vi "Close Sessions.vi"(8 "error in":errorcluster, 11 "session reservation in":refnum<class "Session Reservation.lvclass">) -> (0 "error out":errorcluster, 3 "session reservation out":refnum<class "Session Reservation.lvclass">)   [LabVIEW 2020, in "MeasurementLink Session Management.lvlib" / "Session Reservation.lvclass"]
doc: "Closes all instrument sessions that were created with the session reservation."
uses:
  Session Reservation.lvclass
  Session Reservation.lvclass/Session Reservation.ctl
  MeasurementLink Instrument/IInstrument/IInstrument.lvclass
  MeasurementLink Measurement Server/Helpers/Error Strings Global Internal.vi
  Connection Map/Connection Map.lvclass
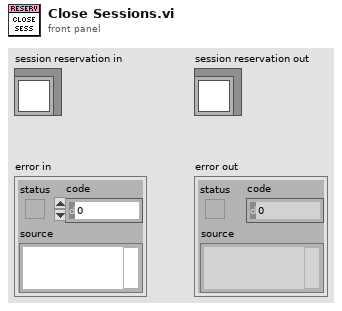
[diagram p1: front panel]
types:
  T1 = typedef "MeasurementLink Session Management.lvlib/Session Reservation.lvclass/Data.ctl" = cluster{"session and driver infos":T2[], "pin or relay names":string[], "connection map":refnum<class "Connection Map.lvclass">, "pin map context":T7, "reservation observer":refnum<class "IReservationObserver.lvclass">, "dvr valid":bool}
  T2 = typedef "MeasurementLink Session Management.lvlib/Session Reservation.lvclass/Session and Driver Info.ctl" = cluster{"session info":T3, "session":variant, "instrument":refnum<class "IInstrument.lvclass">, "initialize and close session behavior":T6}
  T3 = typedef "MeasurementLink Session Management Client.lvlib/ni_measurementlink_sessionmanagement_v1_SessionInformation.ctl" = cluster{"session":T4, "resource_name":string, "channel_list":string, "instrument_type_id":string, "session_exists":bool, "channel_mappings":T5[]}
  T4 = typedef "MeasurementLink Session Management Client.lvlib/nidevice_grpc_Session.ctl" = cluster{"name":string}
  T5 = typedef "MeasurementLink Session Management Client.lvlib/ni_measurementlink_sessionmanagement_v1_ChannelMapping.ctl" = cluster{"pin_or_relay_name":string, "site":i32, "channel":string}
  T6 = typedef "MeasurementLink Instrument.lvlib/IInstrument.lvclass/Initialize and Close Session Behavior.ctl" = enum16{"Create and Close", "Attach and Detach", "Create and Detach", "Attach and Close"}
  T7 = typedef "MeasurementLink Session Management Client.lvlib/ni_measurementlink_PinMapContext.ctl" = cluster{"pin_map_id":string, "sites":i32[]}
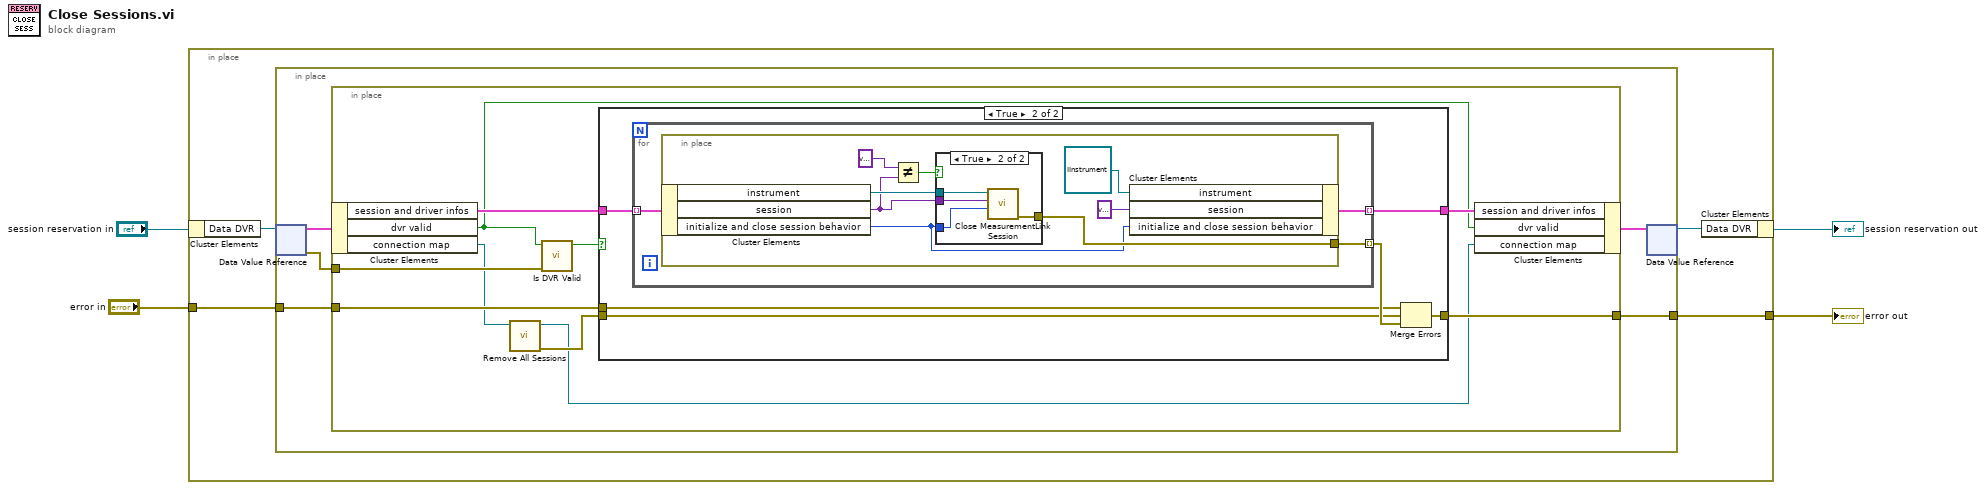
[diagram p0: block diagram]
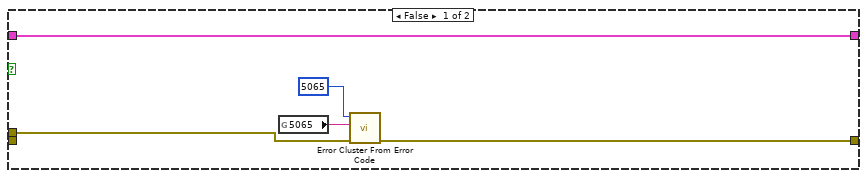
[diagram p2: hidden frame]
diagram:
  n1 = in-place {
    in-place-border: [w6] -> w1
    in-place-border: "error in" -> [w5]
    n2 = in-place-cluster #1("session reservation in") -> ("Data DVR"=w8:refnum<data-value>)
    n3 = in-place {
      in-place-border: [w10] -> w6
      in-place-border: w5 -> [w11]
      n4 = in-place-dvr #2(w8) -> (w12:T1, w13:errorcluster)
      n5 = in-place {
        in-place-border: w13 -> [w23]
        in-place-border: w11 -> [w18]
        in-place-border: [w17] -> w10
        n6 = in-place-cluster #3(w12) -> ("session and driver infos"=w21:T2[], "dvr valid"=w19:bool, "connection map"=w15:refnum<class "Connection Map.lvclass">)
        n7 = call "Remove All Sessions.vi"("connection map in"=w15) -> ("error out"=w16:errorcluster, "connection map out"=w14:refnum<class "Connection Map.lvclass">)  [unwired: 9 in]
        n8 = call "Is DVR Valid.vi"("dvr error in"=w23, "dvr valid"=w19) -> ("dvr valid"=w22:bool)  [unwired: 9 in]
        n9 = case shown="True" w22 {
          tunnel: w21 -> [w28 w34]
          tunnel: [w28 w33] -> w20
          tunnel: w18 -> [w25 w29]
          tunnel: [w24 w32] -> w17
          tunnel: w16 -> [_ w30]
          frame False {
            n10 = global read "Error Strings Global Internal.vi" "5065"() -> (w27:string)
            n11 = call <vilib>:"Error Cluster From Error Code.vi"("error in (no error)"=w25, "error message (\"\")"=w27, "error code (0)"=5065) -> ("error out"=w24:errorcluster)  [unwired: 6 in]
          }
          frame True {
            n12 = for {
              tunnel: w34 -> [w37] mode=indexing
              tunnel: [w36] -> w33 mode=indexing
              tunnel: [w35] -> w31 mode=indexing
              n13 = in-place {
                in-place-border: [w44] -> w35
                n14 = in-place-cluster #4(w37) -> ("instrument"=w43:refnum<class "IInstrument.lvclass">, "session"=w39:variant, "initialize and close session behavior"=w41:T6)
                n15 = Not Equal?(x=variant, y=w39) -> (x != y?=w40:bool)
                n16 = case shown="True" w40 {
                  tunnel: w39 -> [_ w49]
                  tunnel: [_ w48] -> w44
                  tunnel: w43 -> [_ w47]
                  tunnel: w41 -> [_ w46]
                  frame False {
                  }
                  frame True {
                    n17 = call-dynamic "Close MeasurementLink Session.vi"("initialize and close session behavior"=w46, "session in"=w49, "instrument in"=w47) -> ("error out"=w48:errorcluster)  [unwired: 8 in]
                  }
                }
                n18 = in-place-cluster #4("instrument"=refnum<class "IInstrument.lvclass"> refnum, "session"=variant, "initialize and close session behavior"=w41) -> (w36:T2)
              }
            }
            n19 = Merge Errors(w29, w30, w31) -> (w32:errorcluster)
          }
        }
        n20 = in-place-cluster #3("session and driver infos"=w20, "dvr valid"=w19, "connection map"=w14) -> (w9:T1)
      }
      n21 = in-place-dvr #2(w9) -> (w7:refnum<data-value>)  [unwired: 1 out]
    }
    n22 = in-place-cluster #1("Data DVR"=w7) -> (→"session reservation out":refnum<class "Session Reservation.lvclass">)
  }
  "error out" <- w1
